vi "if_v1_v1.vi"() -> ()   [LabVIEW 2009]
panel:
  out "Solutia":dbl=-0.7142857142857143
  in  "b":dbl=5.0
  in  "a":dbl=7.0
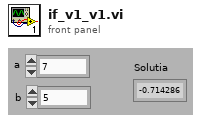
[diagram p1: front panel]
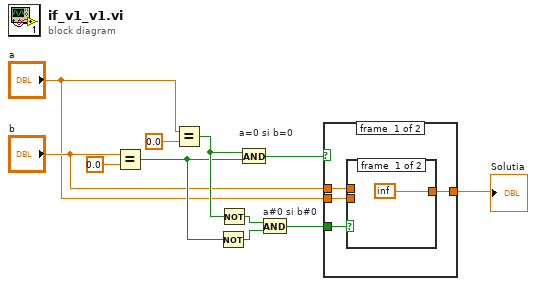
[diagram p0: block diagram]
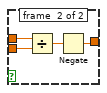
[diagram p2: hidden frame]
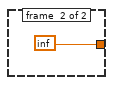
[diagram p3: hidden frame]
diagram:
  n1 = Equal?(x="b", y=0.0) -> (x = y?=w7:bool)
  n2 = Equal?(x="a", y=0.0) -> (x = y?=w9:bool)
  n3 = Not(x=w7) -> (.not. x?=w6:bool)
  n4 = Not(x=w9) -> (.not. x?=w8:bool)
  n5 = And "a=0 si b=0"(x=w9, y=w7) -> (x .and. y?=w5:bool)
  n6 = And "a#0 si b#0"(x=w8, y=w6) -> (x .and. y?=w3:bool)
  n7 = case shown="False" w5 {
    tunnel: [w14 inf] -> w4
    tunnel: w3 -> [w15 _]
    tunnel: "b" -> [w13 _]
    tunnel: "a" -> [w12 _]
    frame #0 {
      n8 = case shown="True" w15 {
        tunnel: [inf w20] -> w14
        tunnel: w13 -> [_ w18]
        tunnel: w12 -> [_ w17]
        frame #0 {
        }
        frame #1 {
          n9 = Divide(x=w18, y=w17) -> (x/y=w19:dbl)
          n10 = Negate(x=w19) -> (-x=w20:dbl)
        }
      }
    }
    frame #1 {
    }
  }
  "Solutia" <- w4
